vi "Controller Test Bench (5).vi"() -> ()   [LabVIEW 2022 SP3]
uses:
  <vilib>/sound2/lvsound2.llb/Sound Data Format.ctl
  <vilib>/Utility/error.llb/DialogType.ctl
  <vilib>/sound2/lvsound2.llb/Sampling Mode.ctl
  <vilib>/Analysis/4window.llb/windowTd.ctl
  <vilib>/DAQmx/read.llb/DAQmx Read (Analog 1D Wfm NChan NSamp).vi
  <vilib>/DAQmx/write.llb/DAQmx Write (Analog 1D DBL 1Chan NSamp).vi
  <vilib>/DAQmx/create/channels.llb/DAQmx Create Channel (AO-Voltage-Basic).vi
  <vilib>/DAQmx/create/channels.llb/DAQmx Create Channel (AI-Acceleration-Accelerometer).vi
  <vilib>/DAQmx/configure/timing.llb/DAQmx Timing (Sample Clock).vi
  <vilib>/DAQmx/miscellaneous.llb/DAQmx Fill In Error Info.vi
  <vilib>/DAQmx/configure/task.llb/DAQmx Configure Logging (TDMS).vi
  <vilib>/measure/maspectr.llb/FFT Spectrum (Mag-Phase) for N Chan.vi
  <vilib>/sound2/lvsound2.llb/Sound Output Set Volume (Single).vi
  <vilib>/sound2/lvsound2.llb/Sound Output Write (DBL Single).vi
  <vilib>/measure/NI_MAPro.lvlib
  <resource>/objmgr/daqmx.rc
  <vilib>/Analysis/NI_AALPro.lvlib
panel:
  out "number of samples written per channel":u32
  in  "Active Control":bool
  in  "Output Noise":bool
  in  "Log Data":bool
  out "Phase 2":cluster{"f0":dbl, "df":dbl, "phase":dbl[]}[](graph)
  out "Mag 2":cluster{"f0":dbl, "df":dbl, "magnitude":dbl[]}[](graph)
  in  "Show FFT":bool
  in  "Save FFT":bool
  in  "Start Acquisition":bool
  in  "Stop":bool
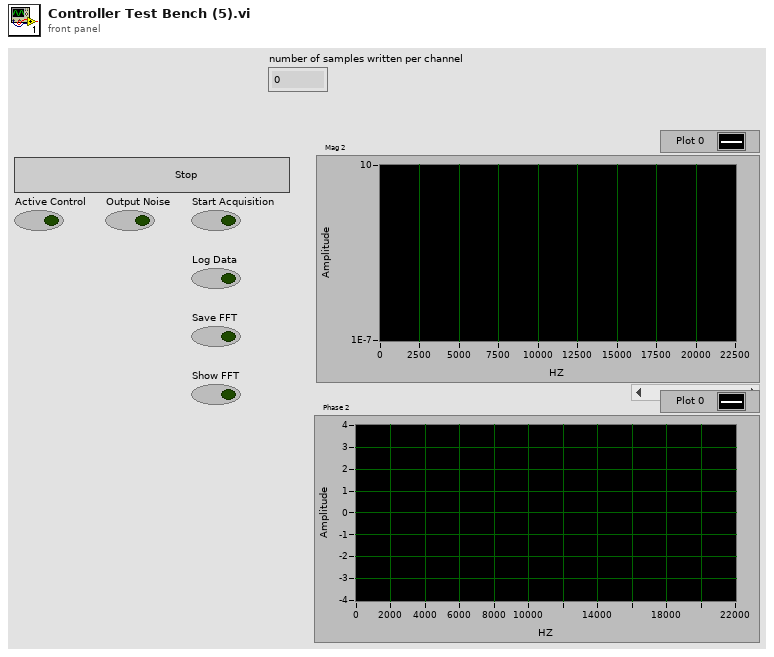
[diagram p1: front panel]
types:
  T1 = typedef "Sampling Mode.ctl" = i32
  T2 = typedef "DialogType.ctl" = u16
  T3 = typedef "Sound Data Format.ctl" = cluster{"sample rate (S/s)":dbl, "number of channels":i32, "bits per sample":i32}
  T4 = typedef "Sound Output Task ID.ctl" = u32
  T5 = typedef "NI_AALPro.lvlib/windowTd.ctl" = u32
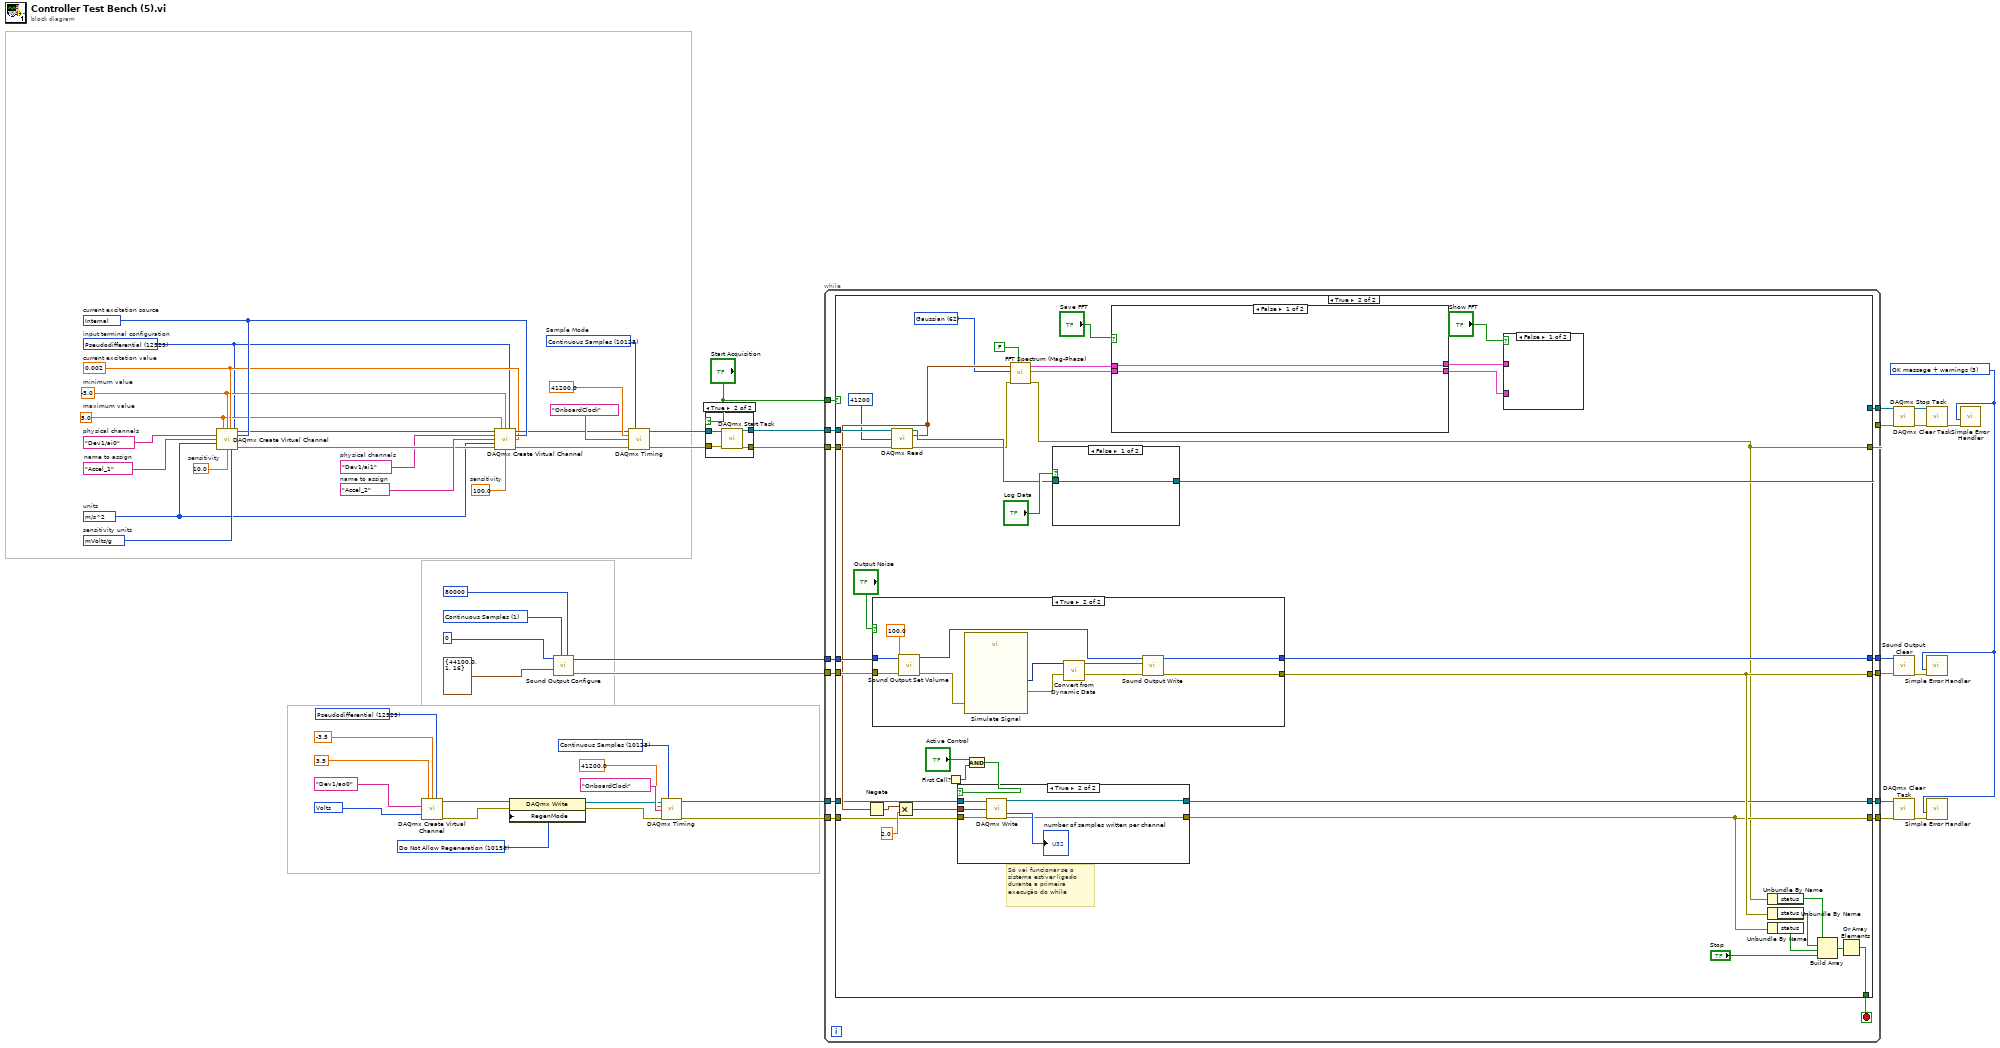
[diagram p0: block diagram]
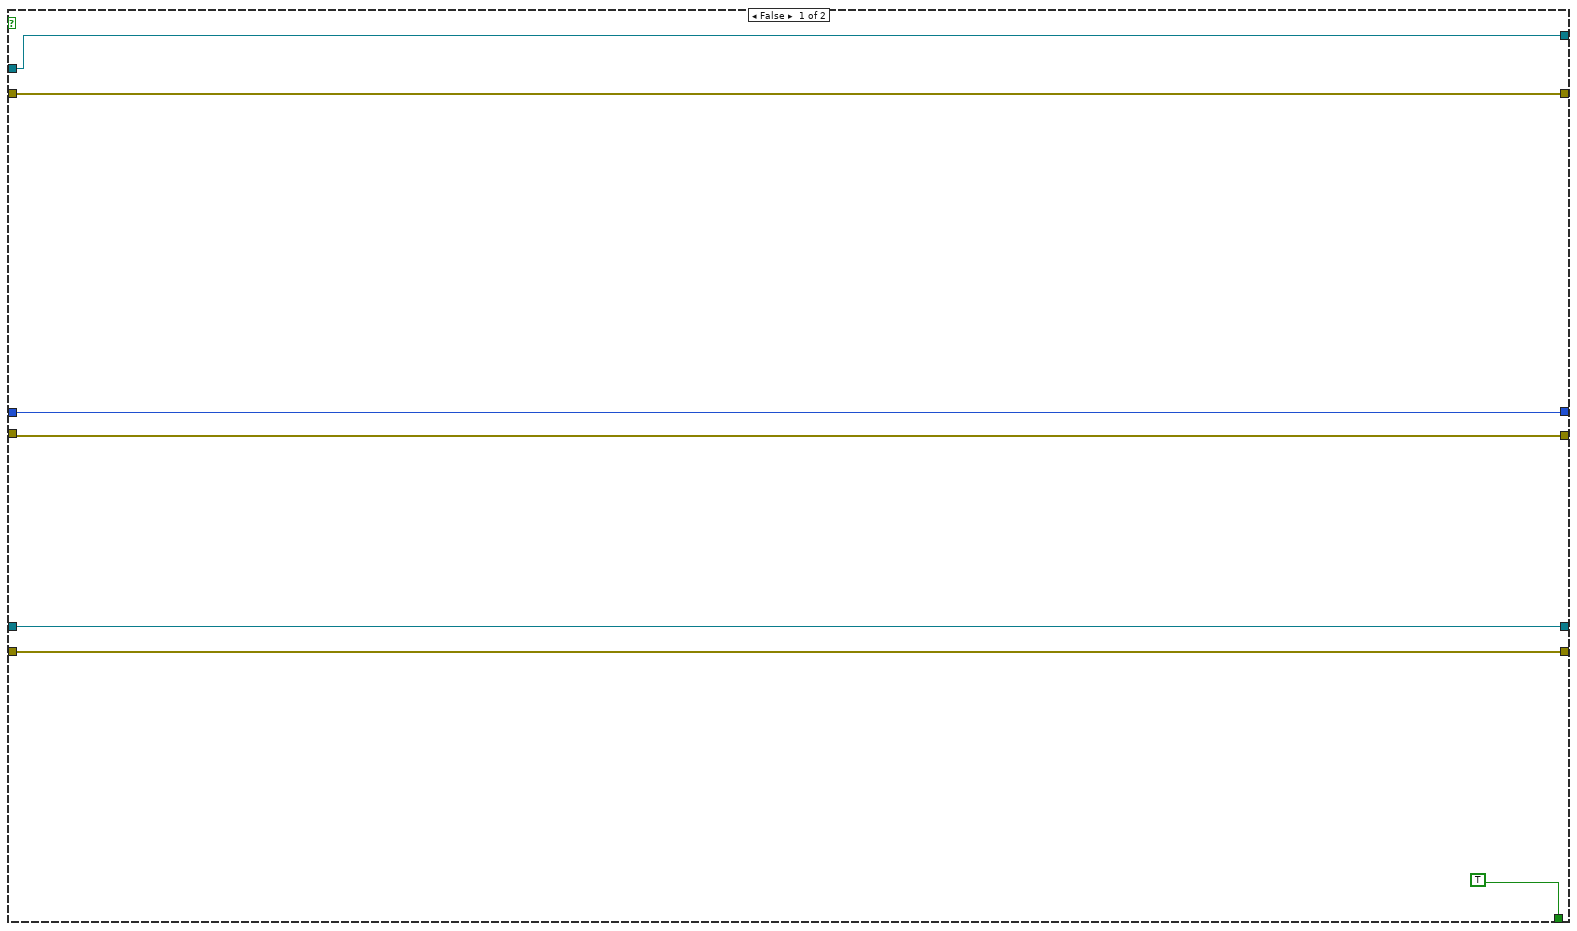
[diagram p3: hidden frame]
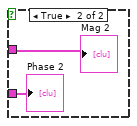
[diagram p6: hidden frame]
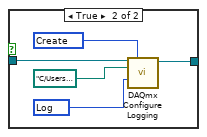
[diagram p8: hidden frame]
diagram:
  w16 = 10123 items=["Finite Samples"=10178, "Continuous Samples"=10123, "Hardware Timed Single Point"=12522] ("sample mode")
  w20 = 12509 items=["mVolts/g"=12509, "Volts/g"=12510]  # sensitivity units
  w21 = 10.0  # sensitivity
  w10 = 0.002  # current excitation value
  w13 = 10200 items=["Internal"=10200, "External"=10167, "None"=10230]  # current excitation source
  w3 = tag "Dev1/ai0"  # physical channels
  w19 = 10123 items=["Finite Samples"=10178, "Continuous Samples"=10123, "Hardware Timed Single Point"=12522]  # Sample Mode
  w6 = 12529 items=["default"=-1, "RSE"=10083, "NRSE"=10078, "Differential"=10106, "Pseudodifferential"=12529]  # input terminal configuration
  w9 = -5.0  # minimum value
  w8 = 5.0  # maximum value
  w22 = "Accel_1"  # name to assign
  w7 = 12470 items=["g"=10186, "m/s^2"=12470, "in/s^2"=12471, "From Custom Scale"=10065]  # units
  w23 = 100.0  # sensitivity
  w4 = tag "Dev1/ai1"  # physical channels
  w15 = "Accel_2"  # name to assign
  w24 = T1 1 items=["Finite Samples", "Continuous Samples"] ("sample mode")
  w37 = 10158 items=["Allow Regeneration"=10097, "Do Not Allow Regeneration"=10158] ("RegenMode")
  w27 = T2 3 items=["no dialog", "OK message", "continue or stop message", "OK message + warnings", "continue/stop + warnings"] ("type of dialog (OK msg:1)")
  w53 = 12529 items=["Default"=-1, "RSE"=10083, "Differential"=10106, "Pseudodifferential"=12529] ("output terminal configuration")
  w51 = 10348 items=["Volts"=10348, "From Custom Scale"=10065] ("units")
  n1 = call-poly <vilib>:"DAQmx Create Virtual Channel.vi"("maximum value"=w8, "minimum value"=w9, "input terminal configuration"=w6, "physical channels"=w3, "current excitation source"=w13, "name to assign"=w22, "current excitation value"=w10, "units"=w7, "sensitivity"=w21, "sensitivity units"=w20) -> ("task out"=w5:refnum<k21>, "error out"=w14:errorcluster)  [unwired: 4 in]
  n2 = call-poly <vilib>:"DAQmx Create Virtual Channel.vi"("maximum value"=3.5, "minimum value"=-3.5, "output terminal configuration"=w53, "physical channels"=tag "Dev1/ao0", "units"=w51) -> ("task out"=w34:refnum<k21>, "error out"=w38:errorcluster)  [unwired: 9 in]
  n3 = call-poly <vilib>:"DAQmx Create Virtual Channel.vi"("task in"=w5, "maximum value"=w8, "minimum value"=w9, "input terminal configuration"=w6, "physical channels"=w4, "current excitation source"=w13, "name to assign"=w15, "current excitation value"=w10, "units"=w7, "error in"=w14, "sensitivity"=w23) -> ("task out"=w12:refnum<k21>, "error out"=w11:errorcluster)  [unwired: 3 in]
  n4 = property class="DAQmx Write"(reference=w34, error in=w38, "RegenMode"=w37) -> (reference out=w32:refnum<k21>, error out=w33:errorcluster)
  n5 = call <vilib>:"Sound Output Configure.vi"("number of samples/ch"=80000 ("Number of Samples/ch"), "sample mode"=w24, "sound format"=T3 {"sample rate (S/s)"=44100.0, "number of channels"=1, "bits per sample"=16} ("Sound Format"), "device ID"=u32 0 ("Device ID")) -> ("error out"=w26:errorcluster, "task ID"=w25:T4)  [unwired: 6 in]
  n6 = call-poly <vilib>:"DAQmx Timing.vi"("task/channels in"=w12, "sample mode"=w19, "rate"=41200.0 ("Sample Rate"), "source"=tag "OnboardClock" ("Sample Clock Source"), "error in"=w11) -> ("task out"=w1:refnum<k21>, "error out"=w2:errorcluster)  [unwired: 9 in]
  n7 = call-poly <vilib>:"DAQmx Timing.vi"("task/channels in"=w32, "sample mode"=w16, "rate"=41200.0 ("Sample Rate"), "source"=tag "OnboardClock" ("Sample Clock Source"), "error in"=w33) -> ("task out"=w36:refnum<k21>, "error out"=w35:errorcluster)  [unwired: 9 in]
  n8 = case shown="True" "Start Acquisition" {
    tunnel: w2 -> [w59 w64]
    tunnel: w1 -> [w60 w63]
    tunnel: [w60 w62] -> w50
    tunnel: [w59 w61] -> w49
    frame False {
    }
    frame True {
      n9 = call <vilib>:"DAQmx Start Task.vi"("task/channels in"=w63, "error in"=w64) -> ("task out"=w62:refnum<k21>, "error out"=w61:errorcluster)  [unwired: 12 in]
    }
  }
  n10 = while {
    tunnel: w26 -> [w78]
    tunnel: w25 -> [w76]
    tunnel: w50 -> [w75]
    tunnel: w49 -> [w74]
    tunnel: [w70] -> w45
    tunnel: [w73] -> w44
    tunnel: [w71] -> w43
    tunnel: [w72] -> w42
    tunnel: w36 -> [w69]
    tunnel: w35 -> [w68]
    tunnel: [w66] -> w31
    tunnel: [w67] -> w30
    tunnel: "Start Acquisition" -> [w65]
    stop <- w77 stop-if-true
    n11 = case shown="True" w65 {
      tunnel: w78 -> [w82 w123]
      tunnel: [TRUE w122] -> w77
      tunnel: w76 -> [w83 w121]
      tunnel: w75 -> [w85 w120]
      tunnel: w74 -> [w84 w119]
      tunnel: [w85 w116] -> w73
      tunnel: [w83 w115] -> w72
      tunnel: [w82 w112] -> w71
      tunnel: [w84 w88] -> w70
      tunnel: w69 -> [w81 w95]
      tunnel: w68 -> [w80 w93]
      tunnel: [w81 w92] -> w67
      tunnel: [w80 w91] -> w66
      frame False {
      }
      frame True {
        w87 = T5 62 items=["Rectangle"=0, "Hanning"=1, "Hamming"=2, "Blackman-Harris"=3, "Exact Blackman"=4, "Blackman"=5, "Flat Top"=6, "4 Term B-Harris "=7, "7 Term B-Harris"=8, "Low Sidelobe"=9, "Blackman Nuttall"=11, "Triangle"=30, "Bartlett-Hanning"=31, "Bohman"=32, "Parzen"=33, "Welch"=34, "Kaiser"=60, "Dolph-Chebyshev"=61, "Gaussian"=62] ("window")
        # "Só vai funcionar se o sistema estiver ligado durante a primeira execução do while"
        n12 = case shown="True" "Output Noise" {
          tunnel: w123 -> [w138 w143]
          tunnel: w121 -> [w139 w144]
          tunnel: [w139 w146] -> w115
          tunnel: [w138 w145] -> w112
          frame False {
          }
          frame True {
            n13 = call-poly <vilib>:"Sound Output Set Volume.vi"("error in (no error)"=w143, "volume"=100.0, "task ID"=w144) -> ("error out"=w142:errorcluster, "task ID out"=w141:T4)  [unwired: 7 in]
            n14 = call "Simulate Signal"("error in (no error)"=w142) -> ("DC with Gaussian Noise"=w149:dynamicdata, "error out"=w148:errorcluster)  [unwired: 13 in]
            n15 = call "Convert from Dynamic Data"("Dynamic Data Type"=w149) -> ("Waveform"=w147:waveform(dbl))  [unwired: 3 in]
            n16 = call-poly <vilib>:"Sound Output Write.vi"("error in (no error)"=w148, "data"=w147, "task ID"=w141) -> ("error out"=w145:errorcluster, "task ID out"=w146:T4)  [unwired: 7 in]
          }
        }
        n17 = call-poly <vilib>:"DAQmx Read.vi"("task/channels in"=w120, "number of samples per channel"=41200, "error in"=w119) -> ("task out"=w117:refnum<k21>, "data"=w101:waveform(dbl)[], "error out"=w89:errorcluster)  [unwired: 10 in]
        n18 = Negate(x=w101) -> (-x=w102:waveform(dbl)[])
        n19 = Multiply(x=w102, y=2.0) -> (x*y=w94:waveform(dbl)[])
        n20 = First Call?() -> (First Call?: T/F=w104:bool)
        n21 = And(x="Active Control", y=w104) -> (x .and. y?=w99:bool)
        n22 = case shown="True" w99 {
          tunnel: w93 -> [w125 w129]
          tunnel: [w124 w126] -> w92
          tunnel: [w125 w127] -> w91
          tunnel: w95 -> [w124 w131]
          tunnel: w94 -> [_ w130]
          frame False {
          }
          frame True {
            n23 = call-poly <vilib>:"DAQmx Write.vi"("task/channels in"=w131, "data"=w130, "error in"=w129) -> ("task out"=w126:refnum<k21>, "number of samples written per channel"=→"number of samples written per channel":u32, "error out"=w127:errorcluster)  [unwired: 10 in]
          }
        }
        n24 = call-poly <vilib>:"FFT Spectrum (Mag-Phase).vi"("restart averaging (F)"=FALSE, "error in (no error)"=w89, "window"=w87, "time signals"=w101) -> ("error out"=w88:errorcluster, "phases"=w107:cluster{"f0":dbl, "df":dbl, "phase":dbl[]}[], "magnitudes"=w108:cluster{"f0":dbl, "df":dbl, "magnitude":dbl[]}[])  [unwired: 3 in, 2 out]
        n25 = case shown="False" "Log Data" {
          tunnel: w117 -> [w150 w152]
          tunnel: [w150 w151] -> w116
          frame False {
          }
          frame True {
            w153 = 15848 items=["Open"=10437, "Open or Create"=15846, "Create or Replace"=15847, "Create"=15848] ("operation")
            w154 = 15844 items=["Off"=10231, "Log"=15844, "Log and Read"=15842] ("logging mode")
            n26 = call-poly <vilib>:"DAQmx Configure Logging.vi"("task/channels in"=w152, "operation"=w153, "file path"=path "C:/Users/LAV-UFSC/Documents/LAV - TCC", "logging mode"=w154) -> ("task out"=w151:refnum<k21>)  [unwired: 10 in, 1 out]
          }
        }
        n27 = case shown="False" "Save FFT" {
          tunnel: w108 -> [w132 w135]
          tunnel: w107 -> [w133 w134]
          tunnel: [w133 w134] -> w106
          tunnel: [w132 w135] -> w103
          frame False {
          }
          frame True {
          }
        }
        n28 = case shown="False" "Show FFT" {
          tunnel: w103 -> [_ w137]
          tunnel: w106 -> [_ w136]
          frame False {
          }
          frame True {
            "Mag 2" <- w137
            "Phase 2" <- w136
          }
        }
        n29 = Unbundle By Name(w88) -> ("status"=w98:bool)
        n30 = Unbundle By Name(w112) -> ("status"=w97:bool)
        n31 = Unbundle By Name(w91) -> ("status"=w96:bool)
        n32 = Build Array(w98, w97, w96, "Stop") -> (w113:bool[])
        n33 = Or Array Elements(Boolean array=w113) -> (logical OR=w122:bool)
      }
    }
  }
  n34 = call <vilib>:"DAQmx Stop Task.vi"("task/channels in"=w44, "error in"=w45) -> ("task out"=w47:refnum<k21>, "error out"=w46:errorcluster)  [unwired: 12 in]
  n35 = call <vilib>:"Sound Output Clear.vi"("error in (no error)"=w43, "task ID"=w42) -> ("error out"=w41:errorcluster)  [unwired: 9 in]
  n36 = call <vilib>:"DAQmx Clear Task.vi"("task in"=w30, "error in"=w31) -> ("error out"=w29:errorcluster)  [unwired: 13 in]
  n37 = call <vilib>:"DAQmx Clear Task.vi"("task in"=w47, "error in"=w46) -> ("error out"=w48:errorcluster)  [unwired: 13 in]
  n38 = call <vilib>:"Simple Error Handler.vi"("type of dialog (OK msg:1)"=w27, "error in (no error)"=w41) -> ()  [unwired: 3 in, 5 out]
  n39 = call <vilib>:"Simple Error Handler.vi"("type of dialog (OK msg:1)"=w27, "error in (no error)"=w29) -> ()  [unwired: 3 in, 5 out]
  n40 = call <vilib>:"Simple Error Handler.vi"("type of dialog (OK msg:1)"=w27, "error in (no error)"=w48) -> ()  [unwired: 3 in, 5 out]
